vi "OpenAvi.vi"(11 "Example Image Path":path) -> (0 "error out":errorcluster, 1 "AVI Refnum (duplicate)":T2, 2 "Sec per Frame":dbl, 3 "Refnum out Image":T1, 5 "Number of Frames For":u32)   [LabVIEW 2015]
uses:
  <vilib>/vision/Avi.llb/IMAQ AVI2 Refnum.ctl
  <vilib>/vision/Image Controls.llb/IMAQ Image.ctl
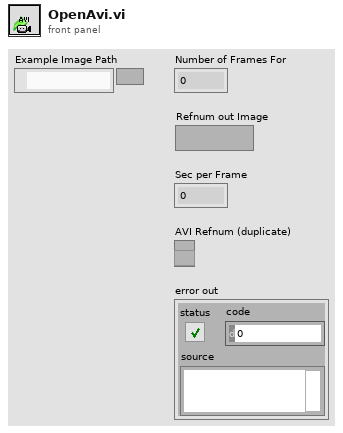
[diagram p1: front panel]
types:
  T1 = typedef "IMAQ Image.ctl" = refnum<image>
  T2 = typedef "IMAQ AVI2 Refnum.ctl" = refnum<k20>
  T3 = typedef "Image Type" = u32
  T4 = cluster{"Width":u32, "Height":u32, "Frames Per Second":u32, "Codec":string, "Has Data":bool}
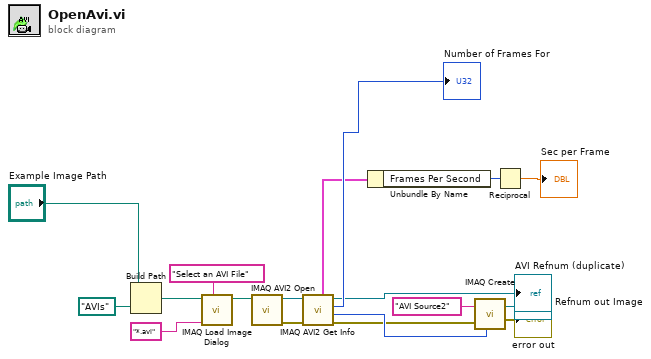
[diagram p0: block diagram]
diagram:
  n1 = Build Path(base path="Example Image Path", name or relative path=path "AVIs") -> (appended path=w15:path)
  n2 = call "IMAQ Load Image Dialog"("Prompt"="Select an AVI File" ("prompt"), "Pattern"="*.avi", "Start Path"=w15) -> ("Path"=w16:path)  [unwired: 6 in, 2 out]
  n3 = call "IMAQ AVI2 Open"("AVI File Path"=w16) -> ("error out"=w3:errorcluster, "AVI Refnum"=w4:T2)  [unwired: 2 in, 7 out]
  n4 = call "IMAQ AVI2 Get Info"("error in (no error)"=w3, "AVI Refnum"=w4) -> ("error out"=w5:errorcluster, "Image Type"=w9:T3, "Number of Frames"=→"Number of Frames For":u32, "AVI Refnum (duplicate)"=→"AVI Refnum (duplicate)":T2, "Frame Data"=w2:T4)  [unwired: 5 out]
  n5 = Unbundle By Name(w2) -> ("Frames Per Second"=w10:u32)
  n6 = call "IMAQ Create"("Image Name"="AVI Source2", "Image Type"=w9, "error in (no error)"=w5) -> ("New Image"=→"Refnum out Image":T1, "error out"=→"error out":errorcluster)  [unwired: 1 in, 1 out]
  n7 = Reciprocal(x=w10) -> (1/x=→"Sec per Frame":dbl)
